vi "Actor Core.vi"(8 "error in":errorcluster, 11 "Temperature Controller in":refnum<class "Temperature Controller.lvclass">) -> (0 "error out":errorcluster, 3 "Actor out":refnum<class "Actor.lvclass">)   [LabVIEW 2021, in "Temperature Controller.lvclass"]
doc: "(<B>Filename</B>: Actor Framework.lvlib:Actor.lvclass:Actor Core.vi)\n\nReceives messages to the actor, reacts to them, and initiates any error handling that may shut the actor down.\n\nDescendant classes may override this VI to append parallel tasks for the actor to complete while it handles messages. Overrides use the Call Parent Method node."
uses:
  Temperature Controller.lvclass
  C:/GitHub/LabActor/Template Module/Template Module.lvclass
  C:/Program Files/National Instruments/LabVIEW 2021/vi.lib/ActorFramework/Actor/Actor.lvclass
  <vilib>/ActorFramework/Actor/Actor.lvclass
  NHMFL_Core/Libraries/Instruments/Temperature Controller Driver/T controller configuration.ctl
  NHMFL_Core/Libraries/Instruments/Temperature Controller/Controls/Control Mode.ctl
  Template Module/Template Module.lvclass/Template Module.ctl
  <vilib>/ActorFramework/Actor/Actor.lvclass/Actor.ctl
  <vilib>/ActorFramework/Message Enqueuer/Message Enqueuer.lvclass/Message Enqueuer.ctl
  Instrument Actor Messages/Send Message Msg/Send Message Msg.lvclass/Send Message Msg.ctl
  Temperature Controller Messages/Set Ramp Msg/Set Ramp Msg.lvclass/Set Ramp Msg.ctl
  Temperature Controller Messages/Set PID Msg/Set PID Msg.lvclass/Set PID Msg.ctl
  Temperature Controller Messages/Set Control Msg/Set Control Msg.lvclass/Set Control Msg.ctl
  Temperature Controller Messages/Set Point Msg/Set Point Msg.lvclass/Set Point Msg.ctl
  Template Module/Read stop event.vi
  <vilib>/ActorFramework/Message Enqueuer/Init from Existing Queue.vi
  <vilib>/ActorFramework/Message Enqueuer/Enqueue.vi
  Instrument Actor Messages/Send Message Msg/Send Message Msg.lvclass
  C:/Program Files/National Instruments/LabVIEW 2021/vi.lib/ActorFramework/Message/Message.lvclass
  Temperature Controller Messages/Set Ramp Msg/Set Ramp Msg.lvclass
  Temperature Controller Messages/Set PID Msg/Set PID Msg.lvclass
  Instrument Actor Messages/Sync Config from Instr Msg/Sync Config from Instr Msg.lvclass
  Temperature Controller Messages/Set Control Msg/Set Control Msg.lvclass
  Temperature Controller Messages/Set Point Msg/Set Point Msg.lvclass
  <vilib>/ActorFramework/Message Priority Queue/Priority Enqueue.vi
  Continuous Recorder Actor/Continuous Recorder Actor.lvclass
  <vilib>/ActorFramework/Message Enqueuer/Message Enqueuer.lvclass
panel:
  in  "Refresh from instrument":bool
  in  "Send Command Button":bool
  in  "Command":string
  out "Name":string
  in  "Configuration":T1={"Record Channels"=["A"], "Record raw signal"=FALSE, "Set point"=0.0, "Record heater"=FALSE, "Ramp rate"=0.0, "P"=0.0, "I"=0.0, "D"=0.0, "Control"=enum."Off", "P manual"=0.0, "Output #"=1}
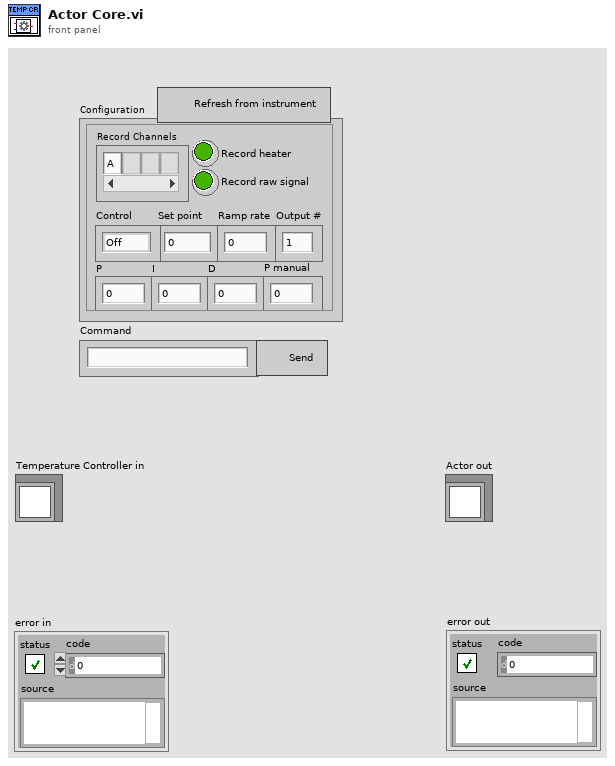
[diagram p1: front panel]
types:
  T1 = typedef "T controller configuration.ctl" = cluster{"Record Channels":string[], "Record raw signal":bool, "Set point":dbl, "Record heater":bool, "Ramp rate":dbl, "P":dbl, "I":dbl, "D":dbl, "Control":T2, "P manual":dbl, "Output #":i32}
  T2 = typedef "Control Mode.ctl" = enum16{"Off", "PID", "Ramp", "Manual", "Table"}
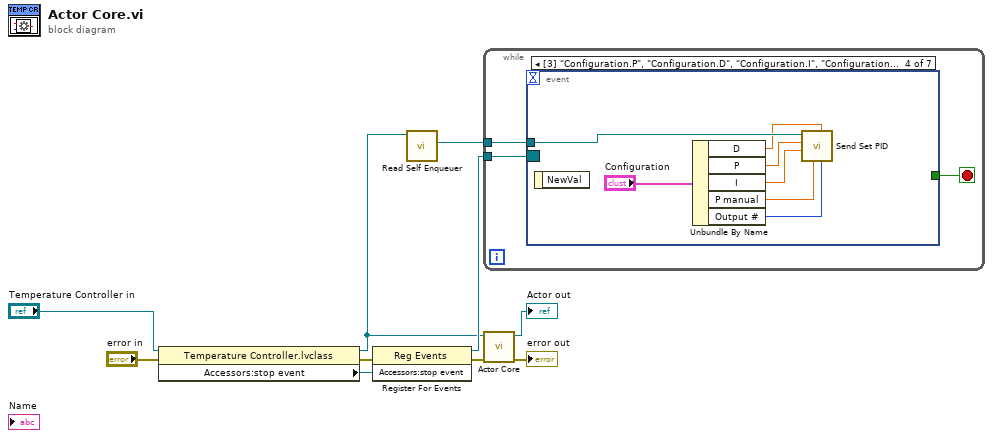
[diagram p0: block diagram]
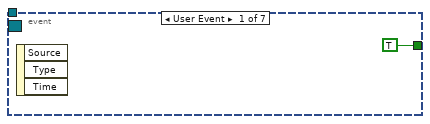
[diagram p2: hidden frame]
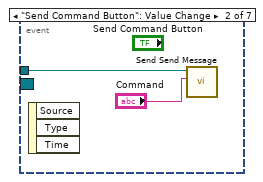
[diagram p3: hidden frame]
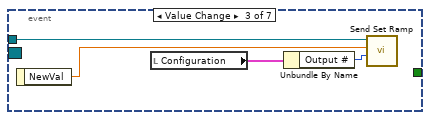
[diagram p4: hidden frame]
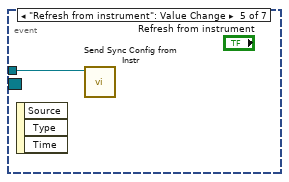
[diagram p5: hidden frame]
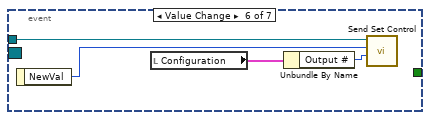
[diagram p6: hidden frame]
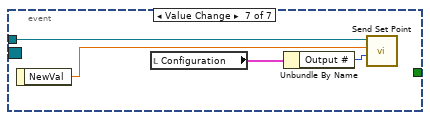
[diagram p7: hidden frame]
diagram:
  n1 = property class="Temperature Controller.lvclass"(reference="Temperature Controller in", error in="error in") -> (reference out=w2:refnum<class "Temperature Controller.lvclass">, error out=w4:errorcluster, "Accessors:stop event"=w6:refnum<user-event>)
  n2 = register-events(error in=w4, w6) -> (reference out=w5:refnum<event-registration>, error out=w3:errorcluster)  [unwired: 1 in]
  n3 = call <vilib>:"Read Self Enqueuer.vi"("Actor"=w2) -> ("Self Enqueuer"=w1:refnum<class "Message Enqueuer.lvclass">)  [unwired: 10 in]
  n4 = while {
    tunnel: w5 -> [w13]
    tunnel: w1 -> [w11]
    stop <- w12 stop-if-true
    n5 = event shown="[3] \"Configuration.P\", \"Configuration.D\", \"Configuration.I\", \"Configuration.P manual\": Value Change" {
      selector: w13 -> [_ _ _ _ _ _ _]
      dyn-events: _ -> [_ _ _ _ _ _ _]
      timeout: _ -> [_ _ _ _ _ _ _]
      tunnel: [TRUE _ _ _ _ _ _] -> w12
      tunnel: w11 -> [_ w16 w20 w23 w28 w31 w36]
      event User Event {
        n6 = event-data() -> ()  [unwired: 1 in, 3 out]
      }
      event "Send Command Button": Value Change {
        n7 = event-data() -> ()  [unwired: 1 in, 3 out]
        n8 = call "Send Send Message.vi"("Message"="Command", "Message Enqueuer"=w16) -> ()  [unwired: 8 in, 2 out]
      }
      event Value Change {
        n9 = event-data() -> ("NewVal"=w19:dbl)  [unwired: 1 in]
        n10 = local read "Configuration"() -> (w18:T1)
        n11 = Unbundle By Name(w18) -> ("Output #"=w17:i32)
        n12 = call "Send Set Ramp.vi"("Output #"=w17, "Ramp rate"=w19, "Message Enqueuer"=w20) -> ()  [unwired: 7 in, 2 out]
      }
      event Value Change {
        n13 = event-data() -> ()  [unwired: 1 in, 1 out]
        n14 = Unbundle By Name("Configuration") -> ("D"=w21:dbl, "P"=w26:dbl, "I"=w25:dbl, "P manual"=w24:dbl, "Output #"=w22:i32)
        n15 = call "Send Set PID.vi"("Output #"=w22, "D"=w21, "P manual"=w24, "I"=w25, "P"=w26, "Message Enqueuer"=w23) -> ()  [unwired: 4 in, 2 out]
      }
      event "Refresh from instrument": Value Change {
        n16 = event-data() -> ()  [unwired: 1 in, 3 out]
        n17 = call "Send Sync Config from Instr.vi"("Message Enqueuer"=w28) -> ()  [unwired: 9 in, 2 out]
      }
      event Value Change {
        n18 = event-data() -> ("NewVal"=w32:T2)  [unwired: 1 in]
        n19 = local read "Configuration"() -> (w30:T1)
        n20 = Unbundle By Name(w30) -> ("Output #"=w29:i32)
        n21 = call "Send Set Control.vi"("Output #"=w29, "Control"=w32, "Message Enqueuer"=w31) -> ()  [unwired: 7 in, 2 out]
      }
      event Value Change {
        n22 = event-data() -> ("NewVal"=w35:dbl)  [unwired: 1 in]
        n23 = local read "Configuration"() -> (w34:T1)
        n24 = Unbundle By Name(w34) -> ("Output #"=w33:i32)
        n25 = call "Send Set Point.vi"("Output #"=w33, "Set point"=w35, "Message Enqueuer"=w36) -> ()  [unwired: 7 in, 2 out]
      }
    }
  }
  n26 = call-parent "Actor Core.vi"("error in"=w3, "Measure Object in"=w2) -> ("error out"=→"error out":errorcluster, "Actor out"=→"Actor out":refnum<class "Actor.lvclass">)  [unwired: 8 in]
